vi "SendSfxUL.vi"(0 "FPGA Reference":refnum<k20>, 1 "Enum":T1, 2 "Pwr Reduction (dB/2)":i8=1, 5 "Tx Payload (Hex)":string, 7 "Tx Freq (Hz)":u32=1, 9 "Freq Offset (Hz)":i32=1, 11 "Error In":errorcluster, 12 "Resp Timeout (ms)":i32 min=0) -> (6 "Send UL OK":bool, 15 "Error Out":errorcluster)   [LabVIEW 2018]
uses:
  Resources_Test/UART/ControlTestSlot.ctl
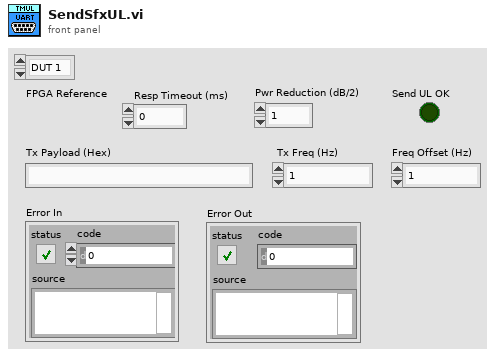
[diagram p1: front panel]
types:
  T1 = typedef "ControlTestSlot.ctl" = enum16{"DUT 1", "DUT 2"}
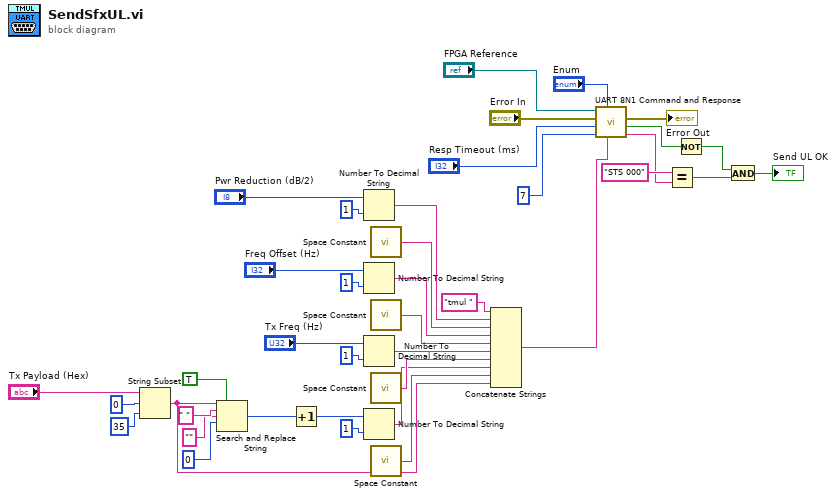
[diagram p0: block diagram]
diagram:
  n1 = String Subset(string="Tx Payload (Hex)", offset (0)=0, length (rest)=35 ("length (rest)")) -> (substring=w15:string)
  n2 = Search and Replace String(replace all?=TRUE ("replace all? (F)"), input string=w15, search string=" ", replace string="" ("replace string (\"\")"), offset=0 ("offset (0)")) -> (number of replacements=w10:i32)  [unwired: 3 in, 3 out]
  n3 = Increment(x=w10) -> (x+1=w9:i32)
  n4 = Number To Decimal String(number="Pwr Reduction (dB/2)", width (-)=i16 1) -> (decimal integer string=w28:string)
  n5 = Number To Decimal String(number="Freq Offset (Hz)", width (-)=i16 1) -> (decimal integer string=w26:string)
  n6 = Number To Decimal String(number="Tx Freq (Hz)", width (-)=i16 1) -> (decimal integer string=w24:string)
  n7 = Number To Decimal String(number=w9, width (-)=i16 1) -> (decimal integer string=w16:string)
  n8 = call <vilib>:"Space Constant.vi"() -> ("String"=w27:string)
  n9 = call <vilib>:"Space Constant.vi"() -> ("String"=w25:string)
  n10 = call <vilib>:"Space Constant.vi"() -> ("String"=w23:string)
  n11 = call <vilib>:"Space Constant.vi"() -> ("String"=w19:string)
  n12 = Concatenate Strings("tmul " ("Text to Send"), w28, w27, w26, w25, w24, w23, w16, w19, w15) -> (w5:string)
  n13 = call "UART 8N1 Command and Response.vi"("Text to Send"=w5, "Active Dut"="Enum", "Response Size (char)"=u32 7, "Response Timeout (ms)"="Resp Timeout (ms)", "Error In"="Error In", "FPGA VI Reference In"="FPGA Reference") -> ("Received Text"=w1:string, "Timeout Flag"=w2:bool, "Error Out"=→"Error Out":errorcluster)  [unwired: 1 in, 2 out]
  n14 = Equal?(x="STS 000" ("y"), y=w1) -> (x = y?=w37:bool)
  n15 = Not(x=w2) -> (.not. x?=w39:bool)
  n16 = And(x=w39, y=w37) -> (x .and. y?=→"Send UL OK":bool)
